vi "myRIO_BRig_RT_TCP__start_exp.vi"(0 "input_hTCP":refnum<k5>, 3 "input_I_connected_TCP":bool, 11 "input_error":errorcluster) -> (4 "output_hTCP":refnum<k5>, 15 "output_error":errorcluster)   [LabVIEW 2014]
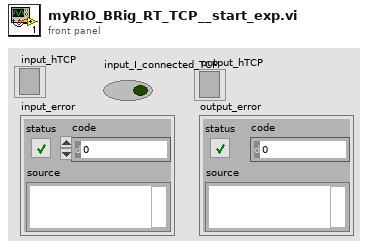
[diagram p1: front panel]
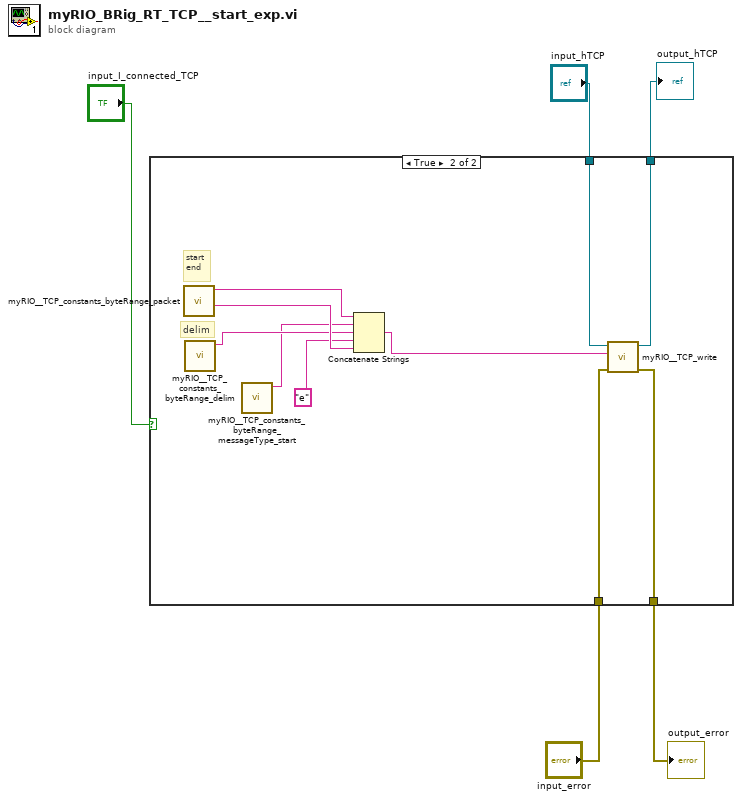
[diagram p0: block diagram]
diagram:
  n1 = case shown="True" "input_I_connected_TCP" {
    tunnel: "input_hTCP" -> [w7 w17]
    tunnel: "input_error" -> [w6 w16]
    tunnel: [w7 w15] -> w3
    tunnel: [w6 w14] -> w2
    frame False {
    }
    frame True {
      # "delim"
      # "start\nend"
      n2 = call "myRIO__TCP_constants_byteRange_packet.vi"() -> ("output_end_char"=w11:string, "output_start_char"=w13:string)  [unwired: 8 in, 2 out]
      n3 = call "myRIO__TCP_constants_byteRange_delim.vi"() -> ("output_delim_char"=w10:string)  [unwired: 10 in, 1 out]
      n4 = call "myRIO__TCP_constants_byteRange_messageType_start.vi"() -> ("output_Start_char"=w9:string)  [unwired: 10 in, 1 out]
      n5 = Concatenate Strings(w13, w9, w10, "e" ("string"), w11) -> (w12:string)
      n6 = call "myRIO__TCP_write.vi"("input_error"=w16, "input_packet"=w12, "input_hTCP"=w17) -> ("output_error"=w14:errorcluster, "output_hTCP"=w15:refnum<k5>)  [unwired: 6 in, 1 out]
    }
  }
  "output_hTCP" <- w3
  "output_error" <- w2
